vi "Get InitializationVI Name.vi"(8 "error in (no error)":errorcluster, 11 "Project XML Editor in":refnum<class "Project XML Editor.lvclass">) -> (0 "error out":errorcluster, 1 "Found ?":bool, 2 "Name out":string, 3 "Project XML Editor out":refnum<class "Project XML Editor.lvclass">)   [LabVIEW 2020, in "LVLIBP CD XML Updater.lvlib" / "Project XML Editor.lvclass"]
uses:
  Project XML Editor.lvclass
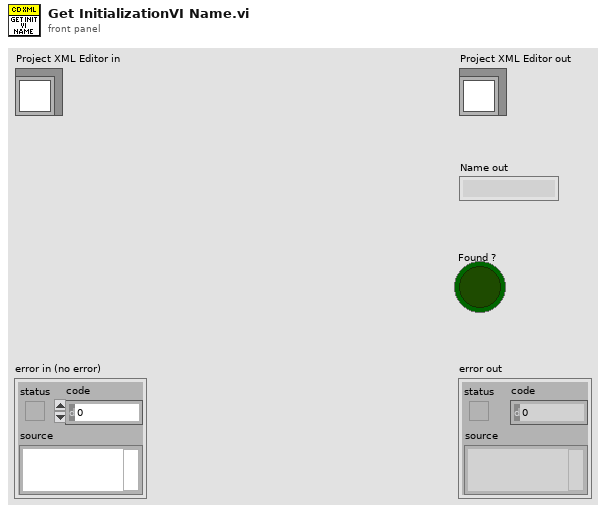
[diagram p1: front panel]
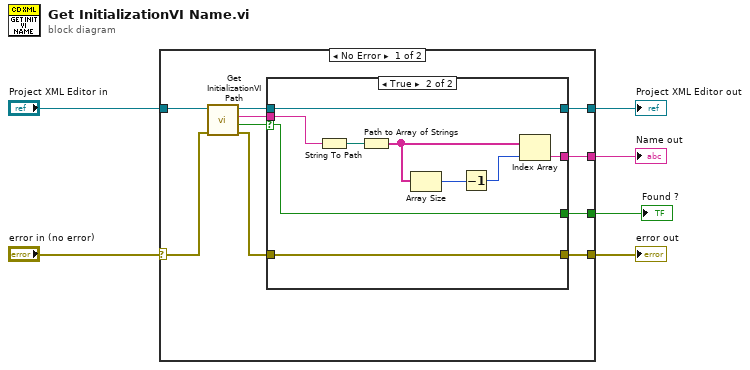
[diagram p0: block diagram]
diagram:
  n1 = case shown="No Error" "error in (no error)" {
    selector: "error in (no error)" -> [w10 w31]
    tunnel: [w8 w31] -> w5
    tunnel: [w11 w30] -> w3
    tunnel: "Project XML Editor in" -> [w16 w30]
    tunnel: [w14 _] -> w2
    tunnel: [w7 _] -> w1
    frame No Error {
      n2 = call "Get InitializationVI Path.vi"("error in (no error)"=w10, "Project XML Editor in"=w16) -> ("error out"=w9:errorcluster, "Found ?"=w13:bool, "Path out"=w15:string, "Project XML Editor out"=w12:refnum<class "Project XML Editor.lvclass">)  [unwired: 6 in]
      n3 = case shown="True" w13 {
        selector: w13 -> [w17 w23]
        tunnel: w15 -> [w19 w29]
        tunnel: [w19 w26] -> w14
        tunnel: w12 -> [w20 w25]
        tunnel: [w20 w25] -> w11
        tunnel: w9 -> [w18 w24]
        tunnel: [w18 w24] -> w8
        tunnel: [w17 w23] -> w7
        frame False {
        }
        frame True {
          n4 = String To Path(string=w29) -> (path=w28:path)
          n5 = Path to Array of Strings(0:w28) -> (2:w27:string[])  [unwired: 1 out]
          n6 = Array Size(array=w27) -> (size(s)=w22:i32)
          n7 = Decrement(x=w22) -> (x-1=w21:i32)
          n8 = Index Array(array=w27, index=w21) -> (element=w26:string)
        }
      }
    }
    frame Error {
    }
  }
  "error out" <- w5
  "Project XML Editor out" <- w3
  "Name out" <- w2
  "Found ?" <- w1
